vi "Configure Acquisition.vi"(0 "VISA resource name":refnum<visa-resource-name>, 5 "Enable Continuous Sweep(F: Disable)":bool, 7 "Trace (1: Trace 1)":i32(ring)=1 items=["Trace 1"=1, "Trace 2"=2, "Trace 3"=3, "Trace 4"=4], 9 "Detector Type(0: Negative Peak)":i32(ring) items=["Negative Peak", "Positive Peak", "Sample", "Average", "Normal"], 11 "error in (no error)":errorcluster) -> (4 "VISA resource name out":refnum<visa-resource-name>, 15 "error out":errorcluster)   [LabVIEW 2022 SP3, in "Agilent N934X Series.lvlib"]
doc: "Configure the acquisition function of the spectrum."
uses:
  <instrlib>/Agilent N934X Series/Agilent N934X Series.lvlib
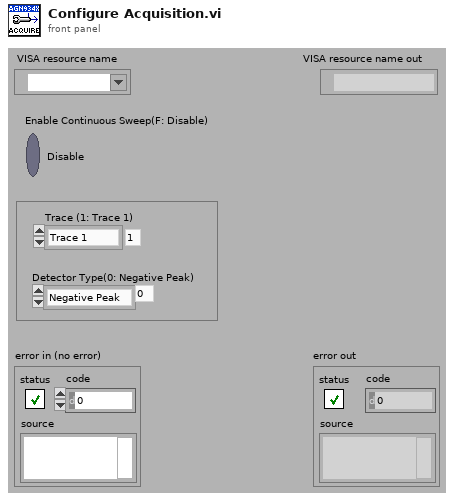
[diagram p1: front panel]
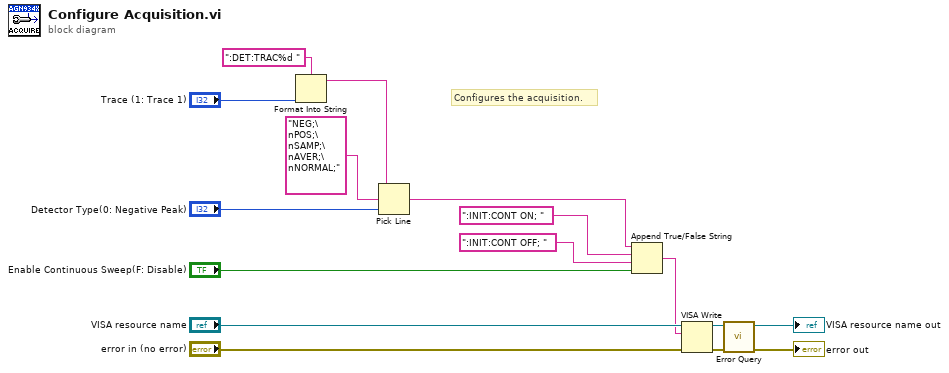
[diagram p0: block diagram]
diagram:
  # "Configures the acquisition."
  n1 = Format Into String(format string=":DET:TRAC%d ", "Trace (1: Trace 1)") -> (resulting string=w7:string)  [unwired: 2 in, 1 out]
  n2 = Pick Line(string ("")=w7, multi-line string="NEG;\nPOS;\nSAMP;\nAVER;\nNORMAL;", line index="Detector Type(0: Negative Peak)") -> (output string=w2:string)
  n3 = Append True/False String(1:"Enable Continuous Sweep(F: Disable)", 2:":INIT:CONT OFF; ", 3:":INIT:CONT ON; ", 4:w2) -> (0:w3:string)
  n4 = VISA Write(VISA resource name="VISA resource name", write buffer=w3, error in (no error)="error in (no error)") -> (VISA resource name out=w16:refnum<visa-resource-name>, error out=w15:errorcluster)  [unwired: 1 out]
  n5 = call <instrlib>:"Error Query.vi"("error in (no error)"=w15, "VISA resource name"=w16) -> ("error out"=→"error out":errorcluster, "VISA resource name out"=→"VISA resource name out":refnum<visa-resource-name>)  [unwired: 6 in, 2 out]
